vi "Go_to_Idle.vi"(8 "error in (no error)":errorcluster, 10 "Nested in":refnum<class "ATM_UI_Controller.lvclass">, 11 "UC_Idle in":refnum<class "UC_Idle.lvclass">) -> (0 "error out":errorcluster, 3 "State out":refnum<class "State Actor.lvclass">)   [LabVIEW 2025, in "User_Console.lvlib" / "UC_Idle.lvclass"]
uses:
  UC_Idle.lvclass
  UC_Idle.lvclass/UC_Idle.ctl
  C:/Users/halstead_rideriver/Documents/Labview_Practice/ATM_Machine_Actor Framework/ATM_ACTORFW/User_Console/User_Console/User_Console.lvclass
  C:/Program Files (x86)/National Instruments/LabVIEW 2025/vi.lib/ni/Actors/State Actor/State Actor/State Actor.lvclass
  C:/Program Files (x86)/National Instruments/LabVIEW 2025/vi.lib/ActorFramework/Actor/Actor.lvclass
  C:/Users/halstead_rideriver/Documents/Labview_Practice/ATM_Machine_Actor Framework/ATM_ACTORFW/User_Console/UC_Idle/UC_Idle.lvclass
  <vilib>/ni/Actors/State Actor/State Actor/State Actor.lvclass
  ATM_UI_Controller/ATM_UI_Controller.lvclass
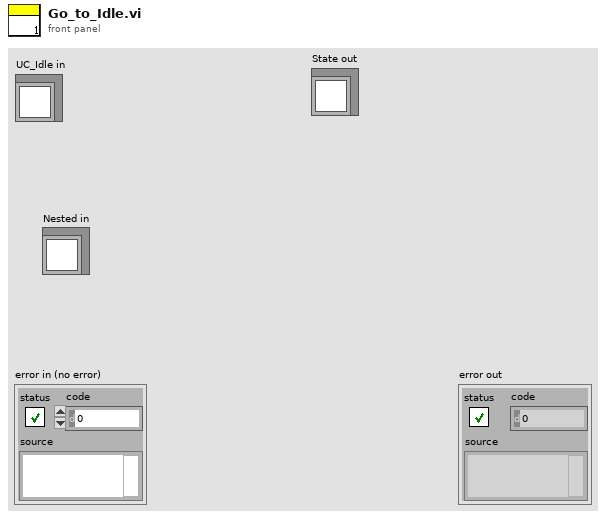
[diagram p1: front panel]
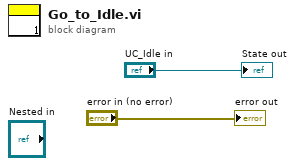
[diagram p0: block diagram]
diagram:
  "error out" <- "error in (no error)"
  "State out" <- "UC_Idle in"
